vi "Initialize Gain.vi"(8 "error in (no error)":errorcluster, 11 "LockinDAQ":refnum<class "LockinDAQ.lvclass">) -> (0 "error out":errorcluster, 3 "LockinDAQ out":refnum<class "LockinDAQ.lvclass">)   [LabVIEW 2016, in "LockinDAQ.lvclass"]
uses:
  LockinDAQ.lvclass
  Instrument.Lockin/Instrument.Lockin.lvclass
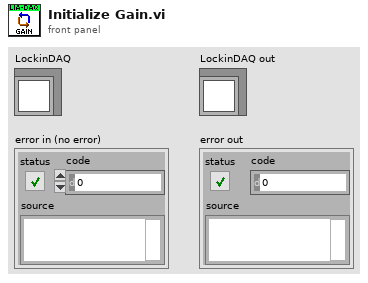
[diagram p1: front panel]
types:
  T1 = typedef "LockinDAQ.lvclass/AO.config-array.ctl" = T2[]
  T2 = typedef "LockinDAQ.lvclass/AO.config-cluster.ctl" = cluster{"AO.channels":tag, "AO.Range":T3, "output terminal configuration":i32, "DAQ Type":T4}
  T3 = typedef "LockinDAQ.lvclass/446xAO-enum.ctl" = enum16{"±0.1 V", "±1.0 V", "±10.0 V"}
  T4 = typedef "LockinDAQ.lvclass/DAQType-enum.ctl" = enum16{"None", "USB 4431", "PXI 446x"}
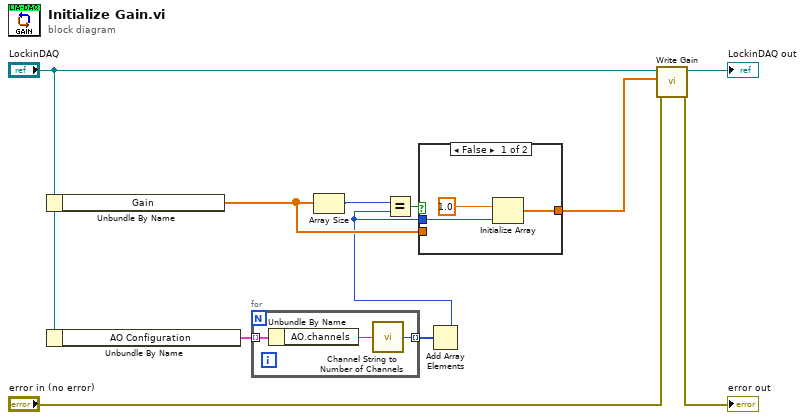
[diagram p0: block diagram]
diagram:
  n1 = Unbundle By Name("LockinDAQ") -> ("Gain"=w10:dbl[])
  n2 = Unbundle By Name("LockinDAQ") -> ("AO Configuration"=w9:T1)
  n3 = for {
    tunnel: w9 -> [w14] mode=indexing
    tunnel: [w12] -> w5 mode=indexing
    n4 = Unbundle By Name(w14) -> ("AO.channels"=w13:tag)
    n5 = call "Channel String to Number of Channels.vi"("Channels String"=w13) -> ("# channels"=w12:i32)  [unwired: 4 in]
  }
  n6 = Array Size(array=w10) -> (size(s)=w6:i32)
  n7 = Add Array Elements(numeric array=w5) -> (sum=w8:i32)
  n8 = Equal?(x=w6, y=w8) -> (x = y?=w7:bool)
  n9 = case shown="False" w7 {
    tunnel: [w15 w18] -> w11
    tunnel: w10 -> [_ w18]
    tunnel: w8 -> [w16 _]
    frame False {
      n10 = Initialize Array(1.0, w16) -> (w15:dbl[])
    }
    frame True {
    }
  }
  n11 = call "Write Gain.vi"("error in (no error)"="error in (no error)", "Gain"=w11, "LockinDAQ"="LockinDAQ") -> ("error out"=→"error out":errorcluster, "LockinDAQ out"=→"LockinDAQ out":refnum<class "LockinDAQ.lvclass">)  [unwired: 7 in]
